vi "Step_Score.vi"(6 "Step_Score":bool, 9 "Step_3":bool, 10 "Step_1":bool, 11 "Ele_At_Pos":bool) -> (0 "Step_3":bool, 1 "Step 1":bool, 2 "Raise_to_Step":bool, 3 "Open_Infeed":bool)   [LabVIEW 2014]
panel:
  in  "Time_Control":dbl=50.0
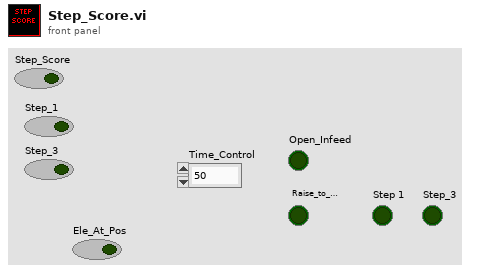
[diagram p1: front panel]
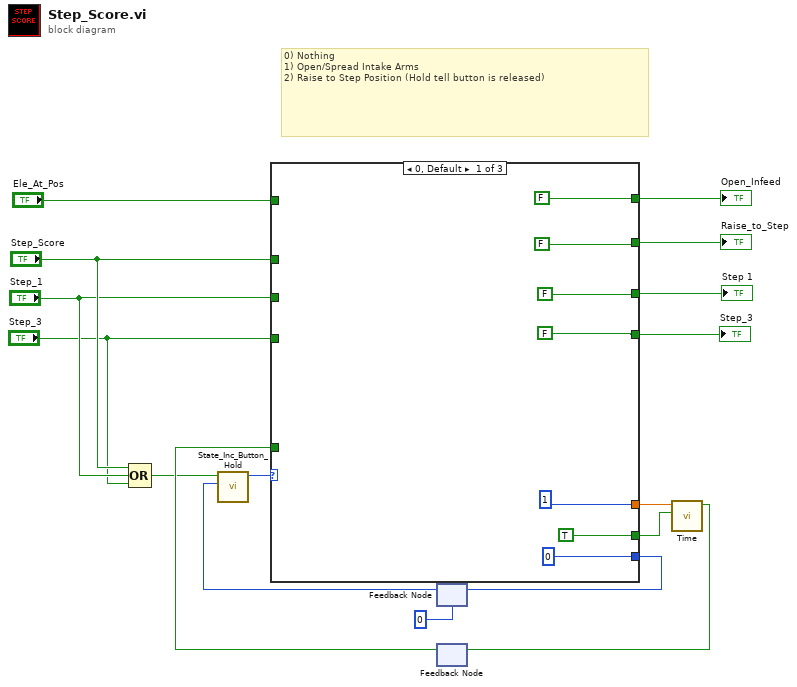
[diagram p0: block diagram]
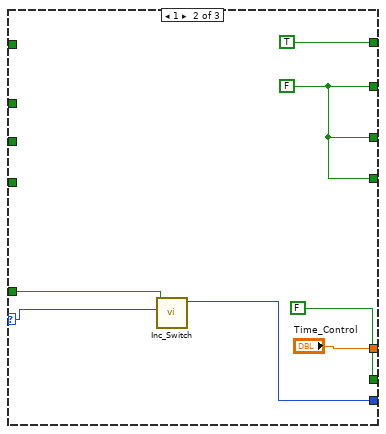
[diagram p2: hidden frame]
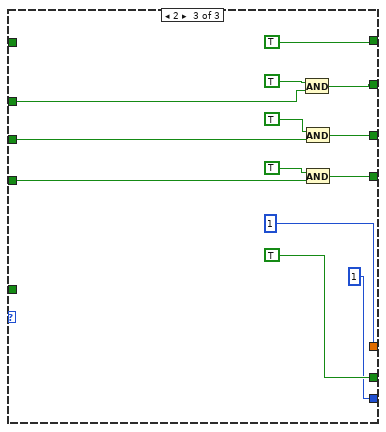
[diagram p3: hidden frame]
diagram:
  # "0) Nothing\n1) Open/Spread Intake Arms\n2) Raise to Step Position (Hold tell button is released)"
  n1 = Compound Arithmetic op=OR("Step_Score", "Step_1", "Step_3") -> (w6:bool)
  n2 = feedback #1(0 ("Numeric out")) -> (w15:i32)
  n3 = call "State_Inc_Button_Hold.vi"("Numeric in"=w15, "Floor_Pickup"=w6) -> ("t"=w17:i32)  [unwired: 9 in]
  n4 = feedback #2() -> (w8:bool)  [unwired: 1 in]
  n5 = case shown="0, Default" w17 {
    selector: w17 -> [_ w30 _]
    tunnel: [0 w31 1 ("Numeric out")] -> w16
    tunnel: [FALSE TRUE TRUE] -> w13
    tunnel: [FALSE w25 w38] -> w12
    tunnel: [1 ("Time_Limit") "Time_Control" 1 ("Time_Limit")] -> w11
    tunnel: [TRUE FALSE TRUE] -> w10
    tunnel: w8 -> [_ w26 _]
    tunnel: "Ele_At_Pos" -> [_ _ _]
    tunnel: [FALSE w25 w35] -> w5
    tunnel: [FALSE w25 w34] -> w4
    tunnel: "Step_Score" -> [_ _ w39]
    tunnel: "Step_1" -> [_ _ w36]
    tunnel: "Step_3" -> [_ _ w32]
    frame 0, Default {
    }
    frame 1 {
      w25 = FALSE
      n6 = call "Inc_Switch.vi"("Numeric in"=w30, "Ele_At_Pos"=w26) -> ("Numeric out"=w31:i32)  [unwired: 9 in]
    }
    frame 2 {
      n7 = And(x=TRUE, y=w39) -> (x .and. y?=w38:bool)
      n8 = And(x=TRUE, y=w36) -> (x .and. y?=w35:bool)
      n9 = And(x=TRUE, y=w32) -> (x .and. y?=w34:bool)
    }
  }
  "Open_Infeed" <- w13
  "Raise_to_Step" <- w12
  "Step 1" <- w5
  "Step_3" <- w4
  n10 = feedback-in #1(w16) -> ()
  n11 = call "Time.vi"("Reset"=w10, "Time_Limit"=w11) -> ("Time_Met"=w9:bool)  [unwired: 9 in]
  n12 = feedback-in #2(w9) -> ()
